vi "gen_freq_array.vi"(0 "Synth Controls":T1={"Channel Settings"=[{"Voltage (Amp.) "=0.0, "Frequency (MHz)"=0.0, "Phase (deg)"=0.0, "Nickname"="Channel 0 D"}, {"Voltage (Amp.) "=0.0, "Frequency (MHz)"=0.0, "Phase (deg)"=0.0, "Nickname"="Channel 0 D"}, {"Voltage (Amp.) "=0.0, "Frequency (MHz)"=0.0, "Phase (deg)"=0.0, "Nickname"="Channel 0 D"}, {"Voltage (Amp.) "=0.0, "Frequency (MHz)"=0.0, "Phase (deg)"=0.0, "Nickname"="Channel 0 D"}], "Active Chans"=[TRUE, FALSE, FALSE, FALSE], "COM Port"="COM5", "Table Mode"={"Initial Freq.(MHz)"=0.0, "FinalFreq"=0.0, "Freq. Step (MHz)"=0.0, "Voltage (Amp.)"=0.0, "Asc. & Desc."=FALSE, "Custom Frequencies"=[], "Custom Amplitude"=[], "Table Mode Switch"=FALSE, "Array Gen"=enum."Auto", "Randomize"=FALSE, "Continuous"=FALSE}} {"Table Mode"."Freq. Step (MHz)" format="%#_9g"; "Table Mode"."FinalFreq" format="%#_9g"; "Table Mode"."Initial Freq.(MHz)" format="%#_9g"; "Channel Settings"."Frequency (MHz)" format="%#_9g"}) -> (7 "Synth Controls Out":T1={"Channel Settings"=[{"Voltage (Amp.) "=0.0, "Frequency (MHz)"=0.0, "Phase (deg)"=0.0, "Nickname"="Channel 0 D"}, {"Voltage (Amp.) "=0.0, "Frequency (MHz)"=0.0, "Phase (deg)"=0.0, "Nickname"="Channel 0 D"}, {"Voltage (Amp.) "=0.0, "Frequency (MHz)"=0.0, "Phase (deg)"=0.0, "Nickname"="Channel 0 D"}, {"Voltage (Amp.) "=0.0, "Frequency (MHz)"=0.0, "Phase (deg)"=0.0, "Nickname"="Channel 0 D"}], "Active Chans"=[TRUE, FALSE, FALSE, FALSE], "COM Port"="COM5", "Table Mode"={"Initial Freq.(MHz)"=0.0, "FinalFreq"=0.0, "Freq. Step (MHz)"=0.0, "Voltage (Amp.)"=0.0, "Asc. & Desc."=FALSE, "Custom Frequencies"=[], "Custom Amplitude"=[], "Table Mode Switch"=FALSE, "Array Gen"=enum."Auto", "Randomize"=FALSE, "Continuous"=FALSE}} {"Table Mode"."Freq. Step (MHz)" format="%#_9g"; "Table Mode"."FinalFreq" format="%#_9g"; "Table Mode"."Initial Freq.(MHz)" format="%#_9g"; "Channel Settings"."Frequency (MHz)" format="%#_9g"}, 9 "Array":dbl[](array[numeric]))   [LabVIEW 2016]
uses:
  Controls/Synth_409b/Synth_controls.ctl
  Controls/Synth_409b/synth_channel.ctl
  Controls/Synth_409b/table_mode.ctl
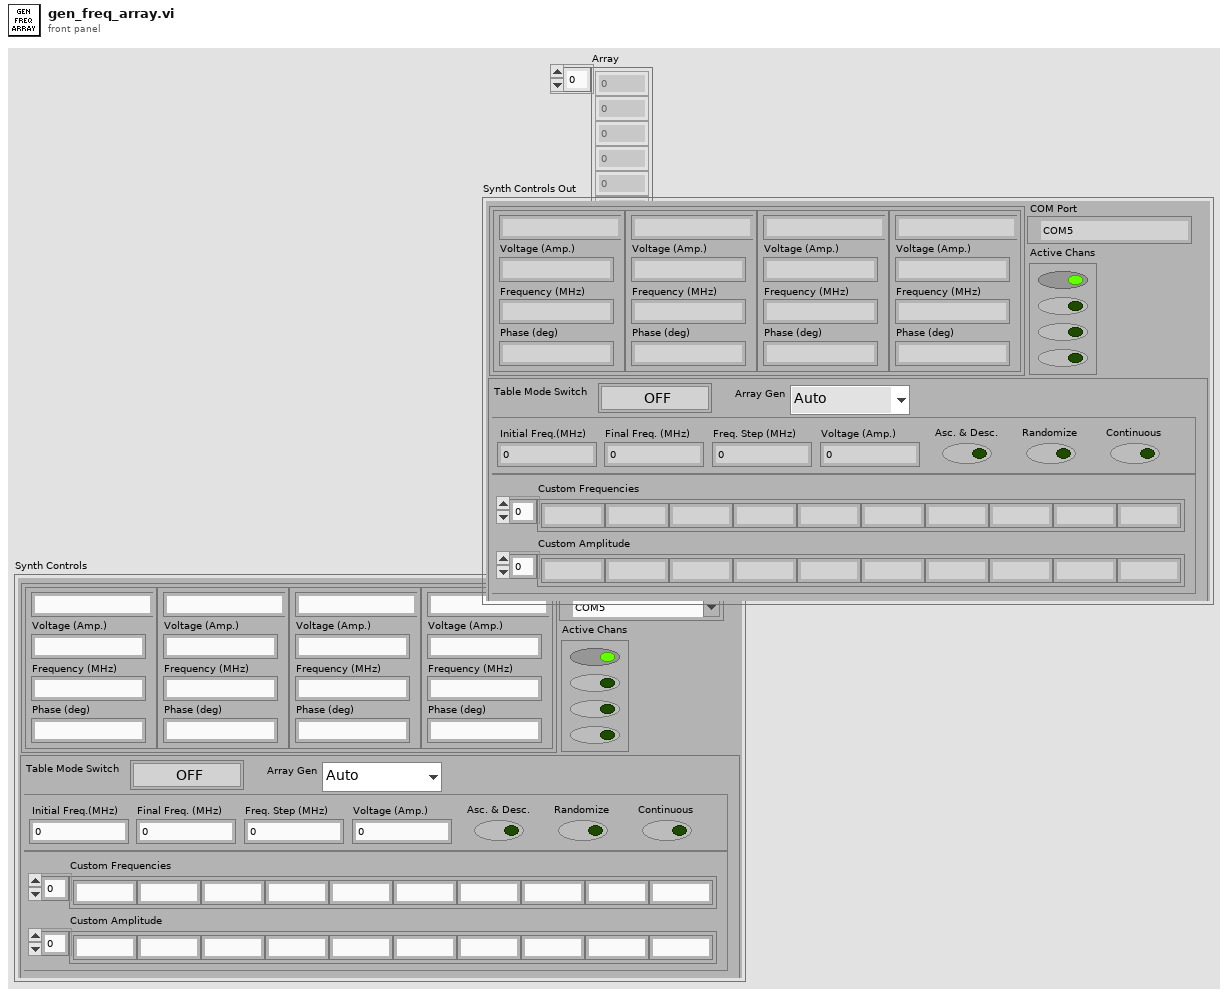
[diagram p1: front panel]
types:
  T1 = typedef "Synth_controls.ctl" = cluster{"Channel Settings":T2[], "Active Chans":bool[], "COM Port":refnum<visa-resource-name>, "Table Mode":T3}
  T2 = typedef "synth_channel.ctl" = cluster{"Voltage (Amp.) ":dbl, "Frequency (MHz)":dbl, "Phase (deg)":dbl, "Nickname":string}
  T3 = typedef "table_mode.ctl" = cluster{"Initial Freq.(MHz)":dbl, "FinalFreq":dbl, "Freq. Step (MHz)":dbl, "Voltage (Amp.)":dbl, "Asc. & Desc.":bool, "Custom Frequencies":dbl[], "Custom Amplitude":dbl[], "Table Mode Switch":bool, "Array Gen":enum16{"Auto", "Custom"}, "Randomize":bool, "Continuous":bool}
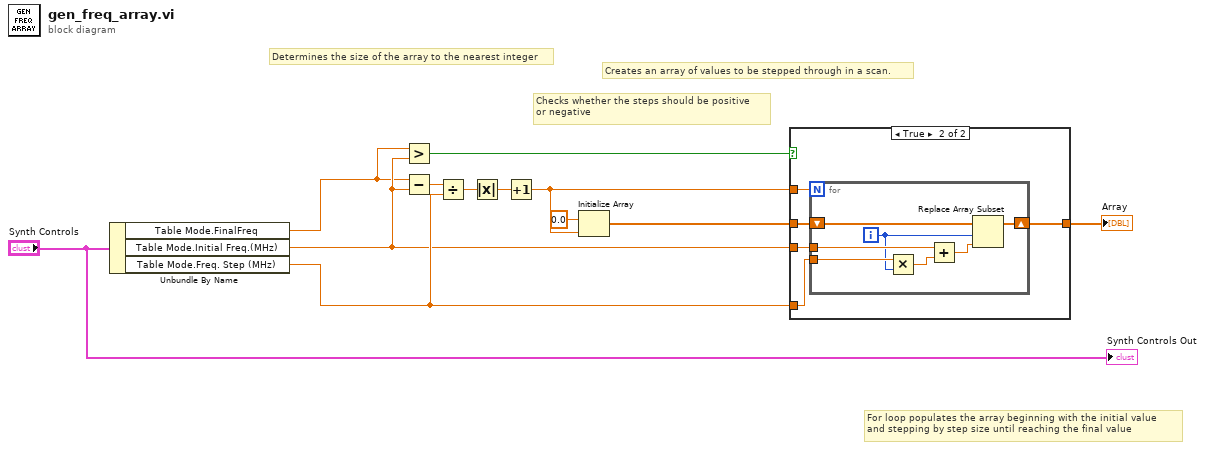
[diagram p0: block diagram]
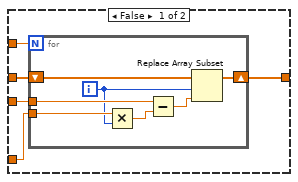
[diagram p2: hidden frame]
diagram:
  # "For loop populates the array beginning with the initial value\nand stepping by step size until reaching the final value"
  # "Determines the size of the array to the nearest integer"
  # "Checks whether the steps should be positive\nor negative"
  # "Creates an array of values to be stepped through in a scan."
  n1 = Unbundle By Name("Synth Controls") -> ("Table Mode.FinalFreq"=w2:dbl, "Table Mode.Initial Freq.(MHz)"=w3:dbl, "Table Mode.Freq. Step (MHz)"=w4:dbl)
  n2 = Greater?(x=w2, y=w3) -> (0:w9:bool)
  n3 = Subtract(x=w2, y=w3) -> (x-y=w12:dbl)
  n4 = Divide(x=w12, y=w4) -> (x/y=w10:dbl)
  n5 = Absolute Value(x=w10) -> (abs(x)=w6:dbl)
  n6 = Increment(x=w6) -> (x+1=w5:dbl)
  n7 = Initialize Array(0.0 ("element"), w5) -> (w8:dbl[])
  n8 = case shown="True" w9 {
    tunnel: w8 -> [w15 w29]
    tunnel: w5 -> [w17 w28]
    tunnel: w4 -> [w14 w27]
    tunnel: w3 -> [w13 w26]
    tunnel: [w16 w25] -> w7
    frame False {
      n9 = for {
        N: w17 -> [_]
        shift-right: [w18] -> w16
        shift-left: w15 -> [w19]
        tunnel: w14 -> [w24]
        tunnel: w13 -> [w23]
        i -> [w21]
        n10 = Multiply(x=w24, y=w21) -> (x*y=w22:dbl)
        n11 = Subtract(x=w23, y=w22) -> (x-y=w20:dbl)
        n12 = Replace Array Subset(array=w19, new element=w20, index=w21) -> (w18:dbl[])
      }
    }
    frame True {
      n13 = for {
        N: w28 -> [_]
        shift-right: [w35] -> w25
        shift-left: w29 -> [w36]
        tunnel: w27 -> [w34]
        tunnel: w26 -> [w33]
        i -> [w30]
        n14 = Multiply(x=w34, y=w30) -> (x*y=w32:dbl)
        n15 = Add(x=w33, y=w32) -> (x+y=w31:dbl)
        n16 = Replace Array Subset(array=w36, new element=w31, index=w30) -> (w35:dbl[])
      }
    }
  }
  "Array" <- w7
  "Synth Controls Out" <- "Synth Controls"
